vi "Find Project Target Item.vi"(8 "target structure name":string, 11 "project":refnum<vi>) -> (0 "found":bool, 3 "TargetItem Refnum":refnum<vi>)   [LabVIEW 2020, in "NI_TargetHelper.lvlib"]
uses:
  <vilib>/TargetSupport/NI_TargetHelper/NI_TargetHelper.lvlib
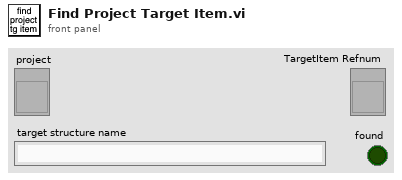
[diagram p1: front panel]
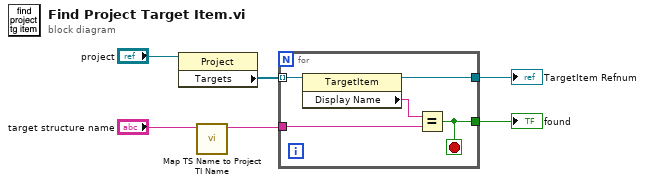
[diagram p0: block diagram]
diagram:
  n1 = property class="Project"(reference="project") -> ("Targets"=w6:refnum<vi>[])  [unwired: 1 in, 2 out]
  n2 = call <vilib>:"Map TS Name to Project TI Name.vi"("target structure name"="target structure name") -> ("project targetitem name"=w5:string)  [unwired: 10 in]
  n3 = for {
    tunnel: w6 -> [w11] mode=indexing
    tunnel: w5 -> [w7]
    tunnel: [w9] -> w2
    tunnel: [w8] -> w1
    stop <- w8 stop-if-true
    n4 = property class="TargetItem"(reference=w11) -> (reference out=w9:refnum<vi>, "Display Name"=w10:string)  [unwired: 1 in, 1 out]
    n5 = Equal?(x=w10, y=w7) -> (x = y?=w8:bool)
  }
  "TargetItem Refnum" <- w2
  "found" <- w1
